vi "Main.vi"(11 "_Template in":refnum<class "_Template.lvclass">) -> (0 "error out":errorcluster, 3 "_Template out":refnum<class "_Template.lvclass">)   [LabVIEW 2025, in "_Template.lvlib" / "_Template.lvclass"]
uses:
  _Template.lvclass
  _Template.lvclass/_Template.ctl
  _Shared/Project Stuff/Project Stuff.lvclass
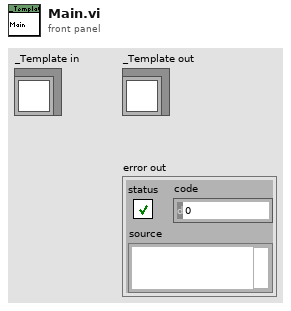
[diagram p1: front panel]
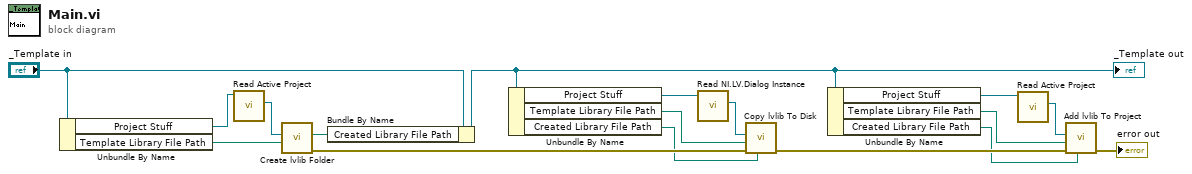
[diagram p0: block diagram]
diagram:
  n1 = Unbundle By Name("_Template in") -> ("Project Stuff"=w7:refnum<class "Project Stuff.lvclass">, "Template Library File Path"=w13:path)
  n2 = call "Read Active Project.vi"("Project Stuff in"=w7) -> ("Active Project"=w6:refnum<vi>)  [unwired: 10 in]
  n3 = call "Create lvlib Folder.vi"("Template Library File Path"=w13, "Active Project"=w6) -> ("error out"=w12:errorcluster, "Created Library File Path"=w14:path)  [unwired: 8 in]
  n4 = Bundle By Name(cluster="_Template in", "Created Library File Path"=w14) -> (w1:refnum<class "_Template.lvclass">)
  "_Template out" <- w1
  n5 = Unbundle By Name(w1) -> ("Project Stuff"=w5:refnum<class "Project Stuff.lvclass">, "Template Library File Path"=w17:path, "Created Library File Path"=w11:path)
  n6 = call "Read NI.LV.Dialog Instance.vi"("Project Stuff in"=w5) -> ("NI.LV.Dialog Instance"=w4:refnum<vi>)  [unwired: 10 in]
  n7 = call "Copy lvlib To Disk.vi"("Created Library File Path"=w11, "error in"=w12, "Template Library File Path"=w17, "NI.LV.Dialog Instance"=w4) -> ("error out"=w16:errorcluster)  [unwired: 7 in]
  n8 = Unbundle By Name(w1) -> ("Project Stuff"=w3:refnum<class "Project Stuff.lvclass">, "Template Library File Path"=w9:path, "Created Library File Path"=w10:path)
  n9 = call "Read Active Project.vi"("Project Stuff in"=w3) -> ("Active Project"=w2:refnum<vi>)  [unwired: 10 in]
  n10 = call "Add lvlib To Project.vi"("Created Library File Path"=w10, "error in"=w16, "Template Library File Path"=w9, "Active Project"=w2) -> ("error out"=→"error out":errorcluster)  [unwired: 7 in]
